vi "Get Device Names.vi"(8 "error in (no error)":errorcluster) -> (0 "error out":errorcluster, 2 "Alias":string[](array[string]), 3 "Resource":string[](array[string]))   [LabVIEW 2025, in "I2C Bus Monitor UI.lvlib"]
uses:
  <vilib>/nisyscfg/Filter Mode.ctl
  <vilib>/nisyscfg/Close (Resources).vi
  <vilib>/nisyscfg/Close (System).vi
  I2C Bus Monitor UI.lvlib
  <resource>/objmgr/nicriosae.rc
  <vilib>/nisyscfg/nisyscfg.lvlib
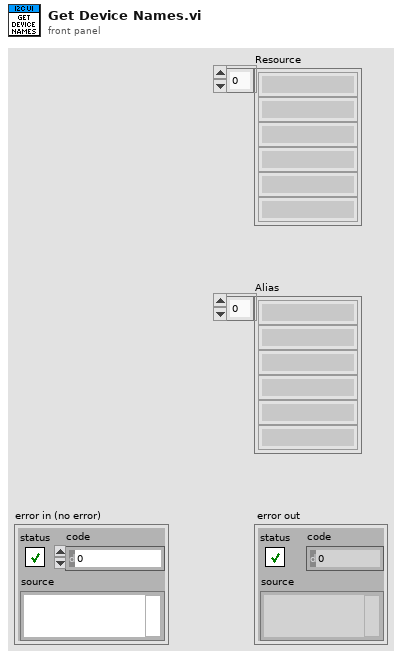
[diagram p1: front panel]
types:
  T1 = typedef "nisyscfg.lvlib/Filter Mode.ctl" = i32
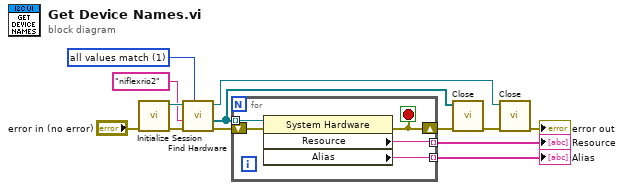
[diagram p0: block diagram]
diagram:
  w11 = T1 1 items=["all values match"=1, "any value matches"=2, "values do not match"=3, "all properties exist"=4] ("filter mode (all values match)")
  n1 = call <vilib>:"Initialize Session.vi"("error in (no error)"="error in (no error)") -> ("error out"=w8:errorcluster, "Session out"=w12:refnum<k21>)  [unwired: 9 in]
  n2 = call <vilib>:"Find Hardware.vi"("Filter Mode (all values match)"=w11, "error in (no error)"=w8, "Experts"="niflexrio2", "Session in"=w12) -> ("error out"=w7:errorcluster, "Resources out"=w3:refnum<k20>[], "Session out"=w13:refnum<k21>)  [unwired: 1 in, 4 out]
  n3 = for {
    tunnel: w3 -> [w18] mode=indexing
    shift-right: [w14] -> w6
    shift-left: w7 -> [w15]
    tunnel: [w17] -> w5 mode=indexing
    tunnel: [w16] -> w4 mode=indexing
    stop <- w14 stop-if-true
    n4 = property class="System Hardware"(reference=w18, error in=w15) -> (error out=w14:errorcluster, "Resource"=w17:string, "Alias"=w16:string)  [unwired: 1 out]
  }
  "Resource" <- w5
  "Alias" <- w4
  n5 = call-poly <vilib>:"Close.vi"("error in (no error)"=w6, "Resources in"=w3) -> ("error out"=w10:errorcluster)  [unwired: 9 in]
  n6 = call-poly <vilib>:"Close.vi"("error in (no error)"=w10, "Session in"=w13) -> ("error out"=→"error out":errorcluster)  [unwired: 9 in]
